vi "CLSUIP_Populate Parent Interface Tree.vi"(6 "Hide Missing (F)":bool, 7 "Parent Class":refnum<vi>, 9 "Class":refnum<vi>, 10 "Parent Interfaces":refnum<vi>[](array[refnum]), 11 "Tree":refnum<vi>) -> (2 "Show Remove Missing?":bool, 3 "Show Legend?":bool)   [LabVIEW 2021]
uses:
  <vilib>/Utility/miscctls.llb/NI.Parent Library Kind.ctl
  c486a13a-825f-4309-9dcc-9f8407b57009.vi
panel:
  in  "Missing Interface":string="This interface is missing.  Either it could not be found on disk, or an LabVIEW encountered an error trying to load it."
  in  "Interface claims parent class!":string="Interface claims parent class!"
  in  "None selected at this time.":string="None selected at this time."
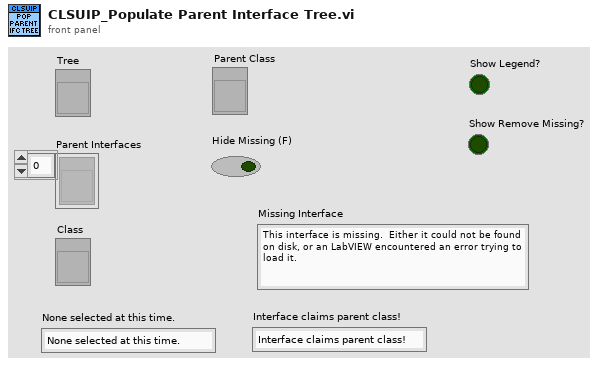
[diagram p1: front panel]
types:
  T1 = typedef "NI.Parent Library Information.ctl" = cluster{"qualified name":string, "localized name":string, "path":path, "parent library kind":T2}
  T2 = typedef "NI.Parent Library Kind.ctl" = enum32{"unknown", "class", "interface"}
  T3 = cluster{"Left Cell String":string, "Child Text":string[], "Child Tag":string, "Item Indent":i32, "Child Only?":bool, "Glyph Index":i32}[]
  T4 = cluster{"Left Cell String":string, "Child Text":string[], "Child Tag":string, "Item Indent":i32, "Child Only?":bool, "Glyph Index":i32}
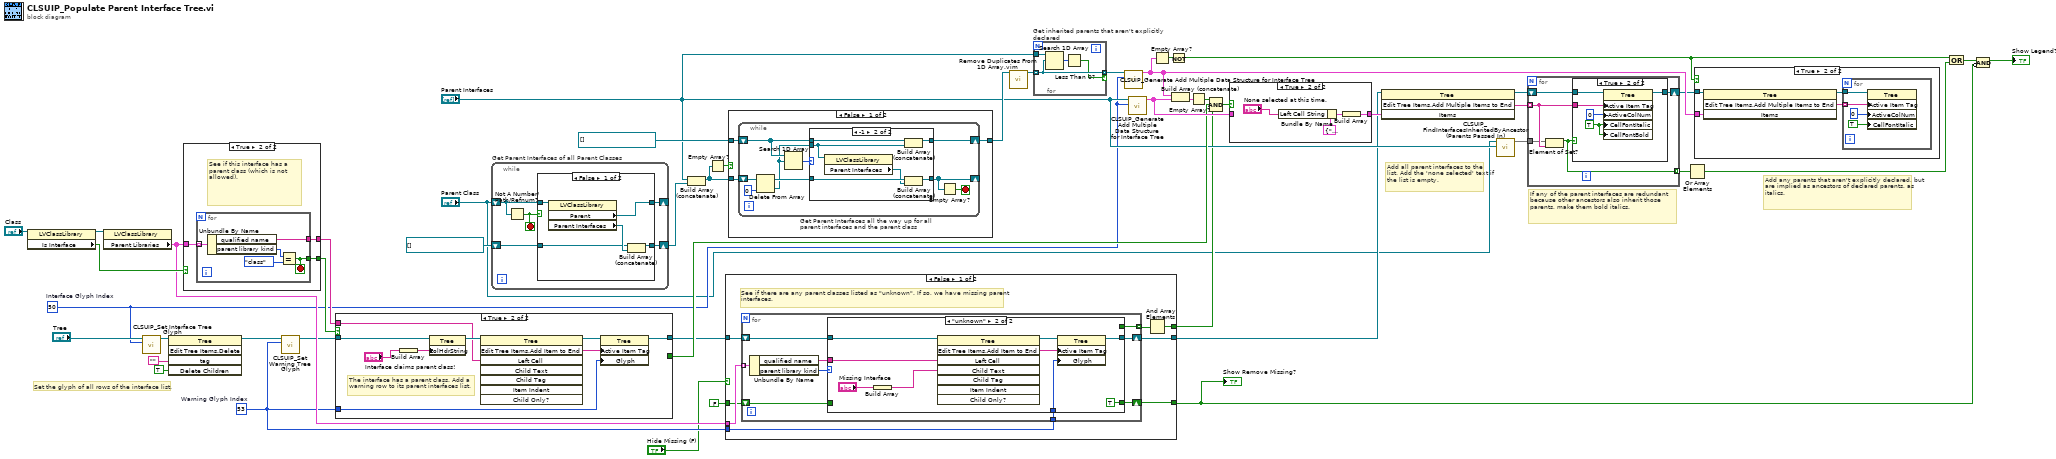
[diagram p0: block diagram]
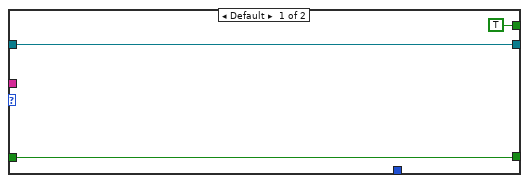
[diagram p2: hidden frame]
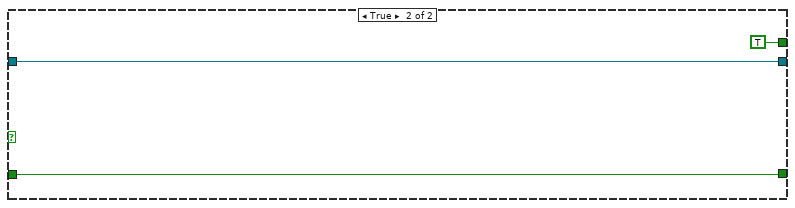
[diagram p3: hidden frame]
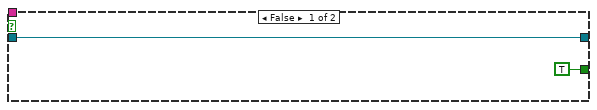
[diagram p4: hidden frame]
diagram:
  w6 = 53  # Warning Glyph Index
  w7 = 50  # Interface Glyph Index
  # "Add any parents that aren't explicitly declared, but are implied as ancestors of declared parents, as italics."
  # "If any of the parent interfaces are redundant because other ancestors also inherit those parents, make them bold italics."
  # "Set the glyph of all rows of the interface list."
  # "Add all parent interfaces to the list. Add the 'none selected' text if the list is empty."
  n1 = property class="LVClassLibrary"(reference="Class") -> (reference out=w11:refnum<vi>, "Is Interface"=w18:bool)  [unwired: 1 in, 1 out]
  n2 = property class="LVClassLibrary"(reference=w11) -> ("Parent Libraries"=w10:T1[])  [unwired: 1 in, 2 out]
  n3 = call <resource>:"CLSUIP_Set Interface Tree Glyph.vi"("Interface Glyph Index (50)"=w7, "TreeControl in"="Tree") -> ("TreeControl out"=w43:refnum<vi>)  [unwired: 8 in, 1 out]
  n4 = invoke class="Tree" method="Edit Tree Items.Delete"(reference=w43, "tag"="", "Delete Children"=TRUE ("Delete Children?")) -> (reference out=w9:refnum<vi>)  [unwired: 2 in, 4 out]
  n5 = case shown="True" w18 {
    tunnel: [_ w50] -> w19
    tunnel: [_ w49] -> w20
    tunnel: w10 -> [_ w48]
    frame False {
    }
    frame True {
      # "See if this interface has a parent class (which is not allowed)."
      n6 = for {
        tunnel: w48 -> [w55] mode=indexing
        tunnel: [w52] -> w50
        tunnel: [w51] -> w49
        stop <- w51 stop-if-true
        n7 = Unbundle By Name(w55) -> ("qualified name"=w52:string, "parent library kind"=w54:T2)
        n8 = Equal?(x=w54, y=NI.Parent_Library_Kind."class") -> (x = y?=w51:bool)
      }
    }
  }
  n9 = call <resource>:"CLSUIP_Set Warning Tree Glyph.vi"("Warning Glyph Index (53)"=w6, "TreeControl in"=w9) -> ("TreeControl out"=w8:refnum<vi>)  [unwired: 8 in, 1 out]
  n10 = case shown="True" w20 {
    tunnel: [w57 w61] -> w13
    tunnel: w8 -> [w57 w59]
    tunnel: w19 -> [_ w62]
    tunnel: [TRUE _] -> w16
    tunnel: w6 -> [_ w58]
    frame False {
    }
    frame True {
      # "The interface has a parent class. Add a warning row to its parent interfaces list."
      n11 = Build Array("Interface claims parent class!") -> (w65:string[])
      n12 = property class="Tree"(reference=w59, "ColHdrString"=w65) -> (reference out=w66:refnum<vi>)  [unwired: 1 in, 1 out]
      n13 = invoke class="Tree" method="Edit Tree Items.Add Item to End"(reference=w66, "Left Cell"=w62) -> (reference out=w63:refnum<vi>, "Edit Tree Items:Add Item to End"=w60:string)  [unwired: 6 in, 6 out]
      n14 = property class="Tree"(reference=w63, "Active Item Tag"=w60, "Glyph"=w58) -> (reference out=w61:refnum<vi>)  [unwired: 1 in, 1 out]
    }
  }
  n15 = while "Get Parent Interfaces of all Parent Classes" {
    shift-right: [w67] -> _
    shift-left: "Parent Class" -> [w69]
    shift-right: [w68] -> w38
    shift-left: refnum<vi>[] [] -> [w71]
    stop <- w70 stop-if-true
    n16 = Not A Number/Path/Refnum?(number/path/refnum=w69) -> (NaN/Path/Refnum?=w70:bool)
    n17 = case shown="False" w70 {
      tunnel: w71 -> [w73 w77]
      tunnel: w69 -> [w76 _]
      tunnel: [w72 w77] -> w68
      tunnel: [w75 _] -> w67
      frame False {
        n18 = property class="LVClassLibrary"(reference=w76) -> ("Parent"=w75:refnum<vi>, "Parent Interfaces"=w74:refnum<vi>[])  [unwired: 1 in, 2 out]
        n19 = Build Array (concatenate)(w73, w74) -> (w72:refnum<vi>[])
      }
      frame True {
      }
    }
  }
  n20 = Build Array (concatenate)("Parent Interfaces", w38) -> (w35:refnum<vi>[])
  n21 = Empty Array?(array=w35) -> (empty?=w34:bool)
  n22 = case shown="False" "Hide Missing (F)" {
    tunnel: [w83 w109] -> w14
    tunnel: w13 -> [w84 w109]
    tunnel: [w81 TRUE] -> w12
    tunnel: w10 -> [w85 _]
    tunnel: w6 -> [w82 _]
    tunnel: FALSE -> [w79 w107]
    tunnel: [w78 w107] -> w2
    frame False {
      # "See if there are any parent classes listed as \"unknown\". If so, we have missing parent interfaces."
      n23 = for {
        tunnel: w85 -> [w94] mode=indexing
        shift-right: [w89] -> w83
        shift-left: w84 -> [w92]
        tunnel: w82 -> [w91]
        tunnel: [w88] -> w80 mode=indexing
        shift-right: [w86] -> w78
        shift-left: w79 -> [w87]
        n24 = Unbundle By Name(w94) -> ("qualified name"=w90:string, "parent library kind"=w93:T2)
        n25 = case shown="\"unknown\"" w93 {
          tunnel: w92 -> [w97 w104]
          tunnel: w91 -> [_ w103]
          tunnel: w90 -> [_ w102]
          tunnel: [w97 w101] -> w89
          tunnel: [TRUE _] -> w88
          tunnel: w87 -> [w95 _]
          tunnel: [w95 TRUE] -> w86
          frame Default {
          }
          frame "unknown" {
            n26 = Build Array("Missing Interface") -> (w99:string[])
            n27 = invoke class="Tree" method="Edit Tree Items.Add Item to End"(reference=w104, "Left Cell"=w102, "Child Text"=w99) -> (reference out=w105:refnum<vi>, "Edit Tree Items:Add Item to End"=w106:string)  [unwired: 5 in, 6 out]
            n28 = property class="Tree"(reference=w105, "Active Item Tag"=w106, "Glyph"=w103) -> (reference out=w101:refnum<vi>)  [unwired: 1 in, 1 out]
          }
        }
      }
      n29 = And Array Elements(Boolean array=w80) -> (logical AND=w81:bool)
    }
    frame True {
    }
  }
  "Show Remove Missing?" <- w2
  n30 = case shown="False" w34 {
    tunnel: refnum<vi>[] [] -> [w112 _]
    tunnel: w35 -> [w111 _]
    tunnel: [w110 _] -> w23
    frame False {
      n31 = while "Get Parent Interfaces all the way up for all parent interfaces and the parent class" {
        shift-right: [w114] -> _
        shift-left: w111 -> [w121]
        shift-right: [w115] -> w110
        shift-left: w112 -> [w118]
        stop <- w113 stop-if-true
        n32 = Delete From Array(array=w121, index=0) -> (deleted portion=w116:refnum<vi>, array with subset deleted=w117:refnum<vi>[])  [unwired: 1 in]
        n33 = Search 1D Array(1D array=w118, element=w116) -> (index of element=w119:i32)  [unwired: 1 in]
        n34 = case shown="-1" w119 {
          tunnel: w118 -> [w123 w129]
          tunnel: w117 -> [w122 w125]
          tunnel: w116 -> [_ w127]
          tunnel: [w123 w128] -> w115
          tunnel: [w122 w126] -> w114
          frame Default {
          }
          frame -1 {
            n35 = property class="LVClassLibrary"(reference=w127) -> ("Parent Interfaces"=w124:refnum<vi>[])  [unwired: 1 in, 2 out]
            n36 = Build Array (concatenate)(w129, w127) -> (w128:refnum<vi>[])
            n37 = Build Array (concatenate)(w125, w124) -> (w126:refnum<vi>[])
          }
        }
        n38 = Empty Array?(array=w114) -> (empty?=w113:bool)
      }
    }
    frame True {
    }
  }
  n39 = call "Remove Duplicates From 1D Array.vim"("array"=w23) -> ("array with duplicates removed"=w22:refnum<vi>[])  [unwired: 10 in]
  n40 = for "Get inherited parents that aren't explicitly declared" {
    tunnel: w22 -> [w132] mode=indexing
    tunnel: "Parent Interfaces" -> [w133]
    tunnel: [w132] -> w37 mode=indexing if=w130
    n41 = Search 1D Array(1D array=w133, element=w132) -> (index of element=w131:i32)  [unwired: 1 in]
    n42 = Less Than 0?(x=w131) -> (x < 0?=w130:bool)
  }
  n43 = call <resource>:"CLSUIP_Generate Add Multiple Data Structure for Interface Tree.vi"("Interface Glyph Index"=w7, "Parent Interfaces"=w37) -> ("Add Multiple Data Structure for Tree"=w32:T3)  [unwired: 8 in, 1 out]
  n44 = call <resource>:"CLSUIP_Generate Add Multiple Data Structure for Interface Tree.vi"("Interface Glyph Index"=w7, "Parent Interfaces"="Parent Interfaces") -> ("Add Multiple Data Structure for Tree"=w47:T3)  [unwired: 8 in, 1 out]
  n45 = Empty Array?(array=w32) -> (empty?=w36:bool)
  n46 = Not(x=w36) -> (.not. x?=w24:bool)
  n47 = Build Array (concatenate)(w32, w47) -> (w33:T3)
  n48 = Empty Array?(array=w33) -> (empty?=w46:bool)
  n49 = Compound Arithmetic op=AND(w46, w16, w12) -> (w17:bool)
  n50 = case shown="True" w17 {
    tunnel: w47 -> [w134 _]
    tunnel: [w134 w137] -> w44
    frame False {
    }
    frame True {
      n51 = Bundle By Name(cluster=T4 {"Left Cell String"="", "Child Text"=[], "Child Tag"="", "Item Indent"=0, "Child Only?"=FALSE, "Glyph Index"=0} ("Item"), "Left Cell String"="None selected at this time.") -> (w136:T4)
      n52 = Build Array(w136) -> (w137:T3)
    }
  }
  n53 = invoke on="Invoke Node" class="Tree" method="Edit Tree Items.Add Multiple Items to End"(reference=w14, "Items"=w44) -> (reference out=w31:refnum<vi>, "Edit Tree Items:Add Multiple Items to End"=w30:string[])  [unwired: 2 in, 2 out]
  n54 = call <resource>:"CLSUIP_FindInterfacesInheritedByAncestor (Parents Passed In).vi"("Parent Interfaces"="Parent Interfaces", "Parent Class"="Parent Class") -> ("indirectly inherited interface item IDs"=w29:set{string})  [unwired: 9 in]
  n55 = for {
    tunnel: w30 -> [w142] mode=indexing
    tunnel: w29 -> [w141]
    tunnel: [w140] -> w26 mode=indexing
    shift-right: [w139] -> w28
    shift-left: w31 -> [w143]
    n56 = Element of Set?(10:w142, 11:w141) -> (3:w140:bool)
    n57 = case shown="True" w140 {
      tunnel: w143 -> [w144 w149]
      tunnel: w142 -> [_ w146]
      tunnel: [w144 w145] -> w139
      frame False {
      }
      frame True {
        w147 = TRUE ("Active Cell:Cell Font:Italic")
        n58 = property class="Tree"(reference=w149, "Active Item Tag"=w146, "ActiveColNum"=0 ("Active Cell:Active Column Number"), "CellFontItalic"=w147, "CellFontBold"=w147) -> (reference out=w145:refnum<vi>)  [unwired: 1 in, 1 out]
      }
    }
  }
  n59 = Or Array Elements(Boolean array=w26) -> (logical OR=w25:bool)
  n60 = case shown="True" w24 {
    tunnel: w28 -> [_ w153]
    tunnel: w32 -> [_ w152]
    frame False {
    }
    frame True {
      n61 = invoke on="Invoke Node" class="Tree" method="Edit Tree Items.Add Multiple Items to End"(reference=w153, "Items"=w152) -> (reference out=w151:refnum<vi>, "Edit Tree Items:Add Multiple Items to End"=w150:string[])  [unwired: 2 in, 2 out]
      n62 = for {
        tunnel: w151 -> [w157]
        tunnel: w150 -> [w156] mode=indexing
        n63 = property class="Tree"(reference=w157, "Active Item Tag"=w156, "ActiveColNum"=0 ("Active Cell:Active Column Number"), "CellFontItalic"=TRUE ("Active Cell:Cell Font:Italic")) -> ()  [unwired: 1 in, 2 out]
      }
    }
  }
  n64 = Compound Arithmetic op=OR(w24, w25) -> (w27:bool)
  n65 = Compound Arithmetic op=AND(w27, invert w2) -> (→"Show Legend?":bool)
